vi "DAC Example (B).vi"() -> ()   [LabVIEW 2011]
doc: "Control the Digital/Analog converter with constant values (basic version)."
uses:
  C:/Program Files/Metrohm Autolab/Autolab SDK 1.10/EcoChemie.Autolab.Sdk.dll
  EcoChemie.Autolab.Sdk.dll
panel:
  out "IsConnected":bool
  in  "stop":bool
  out "error out":errorcluster
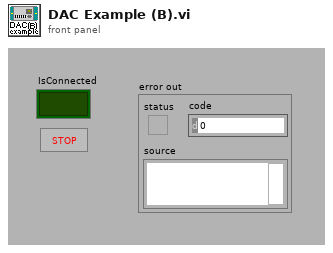
[diagram p1: front panel]
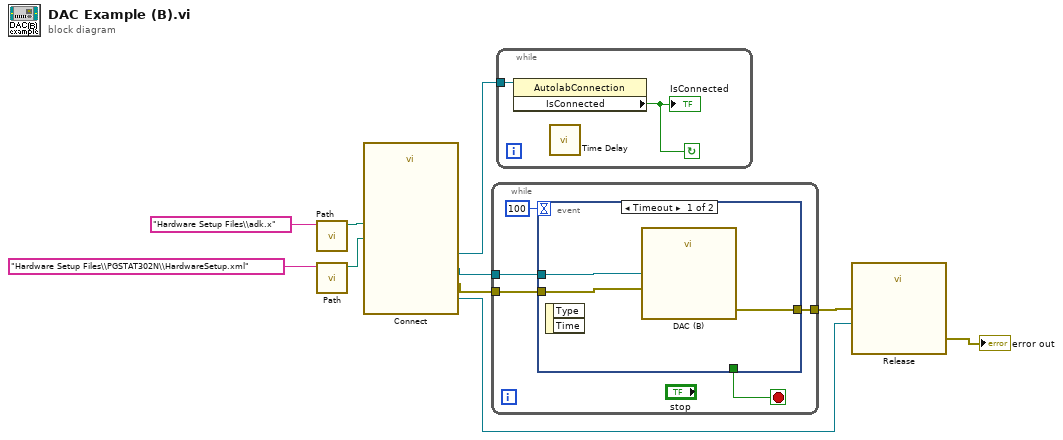
[diagram p0: block diagram]
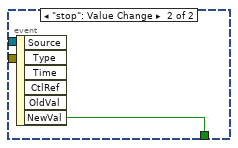
[diagram p2: hidden frame]
diagram:
  n1 = call "Path.vi"("name or relative path"="Hardware Setup Files\\adk.x") -> ("appended path"=w3:path)  [unwired: 10 in]
  n2 = call "Path.vi"("name or relative path"="Hardware Setup Files\\PGSTAT302N\\HardwareSetup.xml") -> ("appended path"=w2:path)  [unwired: 10 in]
  n3 = call "Connect.vi"("Embedded Exe File"=w3, "Hardware Setup File"=w2) -> ("Dac"=w9:refnum<k24>, "AutolabConnection"=w10:refnum<k24>, "instrument"=w7:refnum<k24>, "error out"=w8:errorcluster)  [unwired: 6 in, 4 out]
  n4 = while {
    tunnel: w8 -> [w13]
    tunnel: w9 -> [w14]
    tunnel: [w12] -> w1
    stop <- w11 stop-if-true
    n5 = event shown="[0] Timeout" {
      selector: _ -> [_ _]
      dyn-events: _ -> [_ _]
      timeout: 100 ("Numeric") -> [_ _]
      tunnel: w14 -> [w18 _]
      tunnel: w13 -> [w17 _]
      tunnel: [w16 _] -> w12
      tunnel: [_ w19] -> w11
      event Timeout {
        n6 = event-data() -> ()  [unwired: 1 in, 2 out]
        n7 = call "DAC (B).vi"("error in (no error)"=w17, "Dac"=w18) -> ("error out"=w16:errorcluster)  [unwired: 9 in]
      }
      event "stop": Value Change {
        n8 = event-data() -> ("NewVal"=w19:bool)  [unwired: 1 in, 5 out]
      }
    }
  }
  n9 = while {
    tunnel: w10 -> [w20]
    stop <- w21 continue-if-true
    n10 = property class="AutolabConnection"(reference=w20) -> ("IsConnected"=w21:bool)  [unwired: 1 in, 2 out]
    "IsConnected" <- w21
    n11 = call "Time Delay"() -> ()  [unwired: 11 in, 1 out]
  }
  n12 = call "Release.vi"("error in (no error)"=w1, "Instrument"=w7) -> ("error out"=→"error out":errorcluster)  [unwired: 9 in]
